vi "Decimate (continuous, DBL).vi"(6 "start index":i32, 7 "reset":bool, 8 "error in (no error)":errorcluster, 9 "averaging":bool, 10 "decimating factor":i32=1, 11 "X":dbl[](array[numeric])) -> (0 "error out":errorcluster, 3 "Decimated Array":dbl[](array[numeric]))   [LabVIEW 2017, in "NI_AALPro.lvlib"]
doc: "Continuously decimates the input sequence <B>X</B> by the <B>decimating factor</B> and the <B>averaging</B> Boolean control. Wire data to the <B>X</B> input to determine the polymorphic instance to use or manually select the instance."
uses:
  NI_AALPro.lvlib
  lvanlys.dll
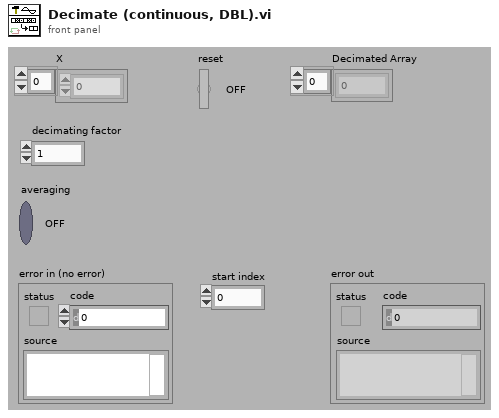
[diagram p1: front panel]
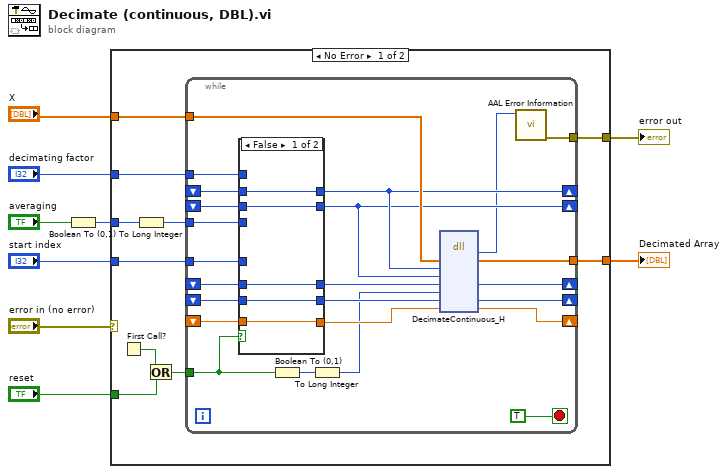
[diagram p0: block diagram]
diagram:
  n1 = Boolean To (0,1)(Boolean="averaging") -> (0, 1=w2:i16)
  n2 = case shown="No Error" "error in (no error)" {
    selector: "error in (no error)" -> [_ w52]
    tunnel: [w17 w52] -> w8
    tunnel: "X" -> [w16 _]
    tunnel: "decimating factor" -> [w15 _]
    tunnel: "start index" -> [w14 _]
    tunnel: "reset" -> [w13 _]
    tunnel: w2 -> [w12 _]
    tunnel: [w10 _] -> w1
    frame No Error {
      n3 = First Call?() -> (First Call?: T/F=w19:bool)
      n4 = To Long Integer(number=w12) -> (32bit integer=w11:i32)
      n5 = Or(x=w19, y=w13) -> (x .or. y?=w18:bool)
      n6 = while {
        tunnel: w16 -> [w42]
        tunnel: w18 -> [w41]
        shift-right: [w39] -> _
        shift-left: _ -> [w38]
        shift-right: [w35] -> _
        shift-left: _ -> [w36]
        tunnel: w15 -> [w40]
        tunnel: w11 -> [w37]
        shift-right: [w34] -> _
        shift-left: _ -> [w33]
        tunnel: w14 -> [w31]
        shift-right: [w29] -> _
        shift-left: _ -> [w27]
        shift-right: [w28] -> _
        shift-left: _ -> [w26]
        tunnel: [w22] -> w17
        tunnel: [w20] -> w10
        stop <- TRUE stop-if-true
        n7 = case shown="False" w41 {
          tunnel: [w48 w51] -> w39
          tunnel: w40 -> [_ w51]
          tunnel: w38 -> [w48 _]
          tunnel: w37 -> [_ w50]
          tunnel: [w47 w50] -> w35
          tunnel: w36 -> [w47 _]
          tunnel: w33 -> [w46 _]
          tunnel: [w46 w49] -> w32
          tunnel: w31 -> [_ w49]
          tunnel: w27 -> [w45 _]
          tunnel: [w45 _] -> w25
          tunnel: w26 -> [w44 _]
          tunnel: [w44 _] -> w24
          frame False {
          }
          frame True {
          }
        }
        n8 = Boolean To (0,1)(Boolean=w41) -> (0, 1=w30:i16)
        n9 = To Long Integer(number=w30) -> (32bit integer=w21:i32)
        n10 = dll-call lib="C:/Program Files/National Instruments/LabVIEW 2017/resource/lvanlys.*" fn="DecimateContinuous_H"("xH"=w42, "decimating factor"=w39, "averaging"=w35, "startIndex"=w32, "reset"=w21, "numSignalInBuffer"=w25, "sumForAverage"=w24) -> (w23:i32, "xH"=w20:dbl[], "startIndex"=w34:i32, "numSignalInBuffer"=w29:i32, "sumForAverage"=w28:dbl)  [unwired: 6 in, 2 out]
        n11 = call "AAL Error Information.vi"("error code"=w23) -> ("error out"=w22:errorcluster)  [unwired: 10 in]
      }
    }
    frame Error {
    }
  }
  "error out" <- w8
  "Decimated Array" <- w1
